vi "ReadFlowMultipleDevices Example.vi"() -> ()   [LabVIEW 2012]
uses:
  BrooksDLL.dll
panel:
  out "S2_2 String":string
  out "S1_2 String":string
  out "S2_1 String":string
  out "S1_1 String":string
  out "S2_2":u8 format="%.0x"
  out "S1_2":u8 format="%.0x"
  out "S2_1":u8 format="%.0x"
  out "S1_1":u8 format="%.0x"
  out "Function Output Comment 2":string
  out "Flow Unit String 2":string
  out "Flow Units 2":u8
  out "Flow 2":sgl format="%.2f"
  out "output param 2":i32
  out "Function Output Comment 1":string
  out "Flow Unit String 1":string
  out "Flow Units 1":u8
  out "Flow 1":sgl format="%.2f"
  out "output param 1":i32
  # "FT01"
  # "FT02"
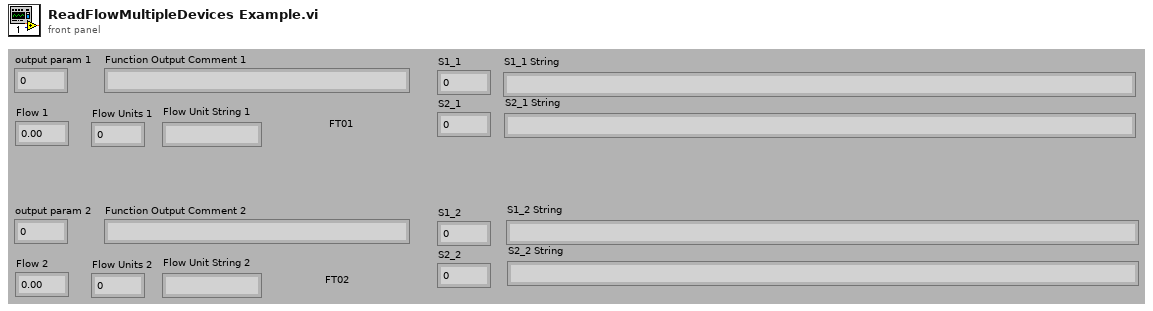
[diagram p1: front panel]
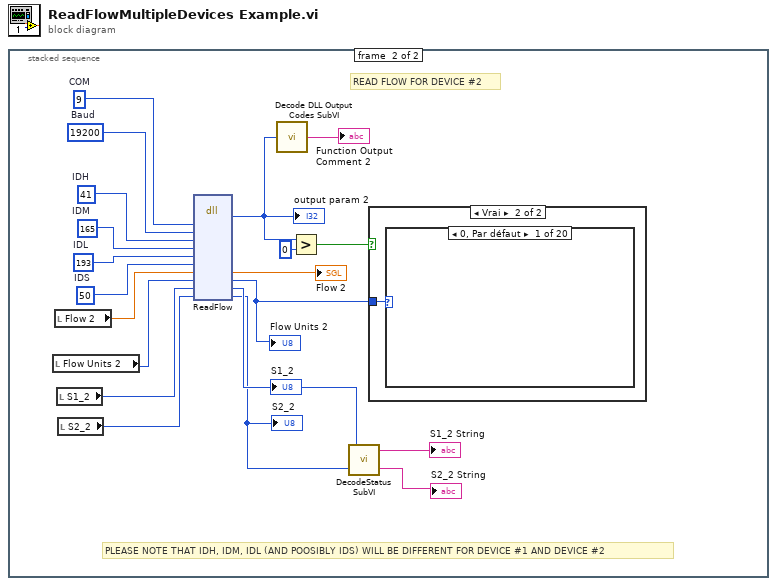
[diagram p0: block diagram]
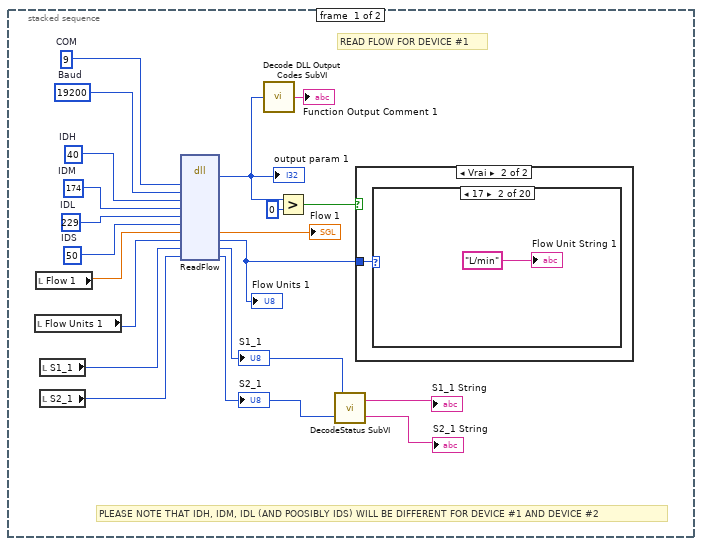
[diagram p2: hidden frame]
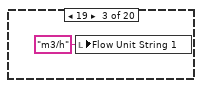
[diagram p5: hidden frame]
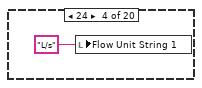
[diagram p6: hidden frame]
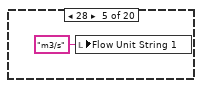
[diagram p7: hidden frame]
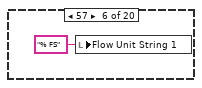
[diagram p8: hidden frame]
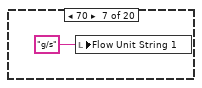
[diagram p9: hidden frame]
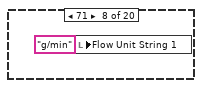
[diagram p10: hidden frame]
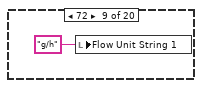
[diagram p11: hidden frame]
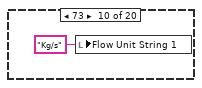
[diagram p12: hidden frame]
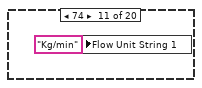
[diagram p13: hidden frame]
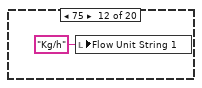
[diagram p14: hidden frame]
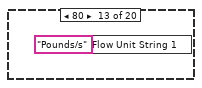
[diagram p15: hidden frame]
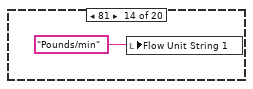
[diagram p16: hidden frame]
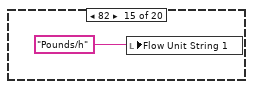
[diagram p17: hidden frame]
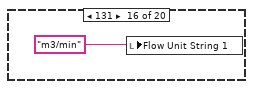
[diagram p18: hidden frame]
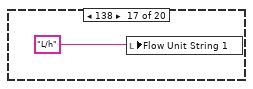
[diagram p19: hidden frame]
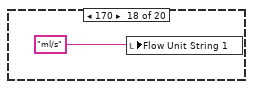
[diagram p20: hidden frame]
diagram:
  n1 = stacked-sequence {
    frame #0 {
      w15 = u8 50  # IDS
      w16 = u8 229  # IDL
      w17 = u8 174  # IDM
      w18 = u8 40  # IDH
      w19 = 19200  # Baud
      w20 = 9  # COM
      # "PLEASE NOTE THAT IDH, IDM, IDL (AND POOSIBLY IDS) WILL BE DIFFERENT FOR DEVICE #1 AND DEVICE #2"
      # "READ FLOW FOR DEVICE #1"
      n2 = local read "Flow Units 1"() -> (w10:u8)
      n3 = local read "Flow 1"() -> (w7:sgl)
      n4 = local read "S1_1"() -> (w6:u8)
      n5 = local read "S2_1"() -> (w5:u8)
      n6 = dll-call lib="C:/Users/Sylvain/Desktop/TopPerm_20150127/drivers/Brooks/S Protocol/BrooksDLL.dll" fn="ReadFlow"("COM"=w20, "Baud"=w19, "IDH"=w18, "IDM"=w17, "IDL"=w16, "IDS"=w15, "Flow"=w7, "FlowUnit"=w10, "S1"=w6, "S2"=w5) -> (w12:i32, "Flow"=→"Flow 1":sgl, "FlowUnit"=w9:u8, "S1"=w4:u8, "S2"=w3:u8)  [unwired: 9 in, 2 out]
      "output param 1" <- w12
      "Flow Units 1" <- w9
      "S1_1" <- w4
      "S2_1" <- w3
      n7 = call "Decode DLL Output Codes SubVI.vi"("Numeric"=w12) -> ("Function Output Comment"=→"Function Output Comment 1":string)
      n8 = Greater?(x=w12, y=0) -> (0:w14:bool)
      n9 = call "DecodeStatus SubVI.vi"("S2"=w3, "S1"=w4) -> ("S2 String"=→"S2_1 String":string, "S1 String"=→"S1_1 String":string)
      n10 = case shown="Vrai" w14 {
        tunnel: w9 -> [_ w21]
        frame False {
        }
        frame True {
          n11 = case shown="17" w21 {
            frame 0, Default {
            }
            frame 17 {
              "Flow Unit String 1" <- "L/min"
            }
            frame 19 {
              n12 = local write "Flow Unit String 1"("m3/h") -> ()
            }
            frame 24 {
              n13 = local write "Flow Unit String 1"("L/s") -> ()
            }
            frame 28 {
              n14 = local write "Flow Unit String 1"("m3/s") -> ()
            }
            frame 57 {
              n15 = local write "Flow Unit String 1"("% FS") -> ()
            }
            frame 70 {
              n16 = local write "Flow Unit String 1"("g/s") -> ()
            }
            frame 71 {
              n17 = local write "Flow Unit String 1"("g/min") -> ()
            }
            frame 72 {
              n18 = local write "Flow Unit String 1"("g/h") -> ()
            }
            frame 73 {
              n19 = local write "Flow Unit String 1"("Kg/s") -> ()
            }
            frame 74 {
              n20 = local write "Flow Unit String 1"("Kg/min") -> ()
            }
            frame 75 {
              n21 = local write "Flow Unit String 1"("Kg/h") -> ()
            }
            frame 80 {
              n22 = local write "Flow Unit String 1"("Pounds/s") -> ()
            }
            frame 81 {
              n23 = local write "Flow Unit String 1"("Pounds/min") -> ()
            }
            frame 82 {
              n24 = local write "Flow Unit String 1"("Pounds/h") -> ()
            }
            frame 131 {
              n25 = local write "Flow Unit String 1"("m3/min") -> ()
            }
            frame 138 {
              n26 = local write "Flow Unit String 1"("L/h") -> ()
            }
            frame 170 {
              n27 = local write "Flow Unit String 1"("ml/s") -> ()
            }
            frame 171 {
              n28 = local write "Flow Unit String 1"("ml/min") -> ()
            }
            frame 172 {
              n29 = local write "Flow Unit String 1"("ml/h") -> ()
            }
          }
        }
      }
    }
    frame #1 {
      w55 = u8 50  # IDS
      w56 = u8 193  # IDL
      w57 = u8 165  # IDM
      w58 = u8 41  # IDH
      w59 = 19200  # Baud
      w60 = 9  # COM
      # "PLEASE NOTE THAT IDH, IDM, IDL (AND POOSIBLY IDS) WILL BE DIFFERENT FOR DEVICE #1 AND DEVICE #2"
      # "READ FLOW FOR DEVICE #2"
      n30 = local read "Flow Units 2"() -> (w48:u8)
      n31 = local read "Flow 2"() -> (w47:sgl)
      n32 = local read "S1_2"() -> (w46:u8)
      n33 = local read "S2_2"() -> (w45:u8)
      n34 = dll-call lib="C:/Users/Sylvain/Desktop/TopPerm_20150127/drivers/Brooks/S Protocol/BrooksDLL.dll" fn="ReadFlow"("COM"=w60, "Baud"=w59, "IDH"=w58, "IDM"=w57, "IDL"=w56, "IDS"=w55, "Flow"=w47, "FlowUnit"=w48, "S1"=w46, "S2"=w45) -> (w51:i32, "Flow"=→"Flow 2":sgl, "FlowUnit"=w49:u8, "S1"=w44:u8, "S2"=w43:u8)  [unwired: 9 in, 2 out]
      "output param 2" <- w51
      "Flow Units 2" <- w49
      "S1_2" <- w44
      "S2_2" <- w43
      n35 = call "Decode DLL Output Codes SubVI.vi"("Numeric"=w51) -> ("Function Output Comment"=→"Function Output Comment 2":string)
      n36 = Greater?(x=w51, y=0) -> (0:w54:bool)
      n37 = call "DecodeStatus SubVI.vi"("S2"=w43, "S1"=w44) -> ("S2 String"=→"S2_2 String":string, "S1 String"=→"S1_2 String":string)
      n38 = case shown="Vrai" w54 {
        tunnel: w49 -> [_ w61]
        frame False {
        }
        frame True {
          n39 = case shown="0, Par défaut" w61 {
            frame 0, Default {
            }
            frame 17 {
              "Flow Unit String 2" <- "L/min"
            }
            frame 19 {
              n40 = local write "Flow Unit String 2"("m3/h") -> ()
            }
            frame 24 {
              n41 = local write "Flow Unit String 2"("L/s") -> ()
            }
            frame 28 {
              n42 = local write "Flow Unit String 2"("m3/s") -> ()
            }
            frame 57 {
              n43 = local write "Flow Unit String 2"("% FS") -> ()
            }
            frame 70 {
              n44 = local write "Flow Unit String 2"("g/s") -> ()
            }
            frame 71 {
              n45 = local write "Flow Unit String 2"("g/min") -> ()
            }
            frame 72 {
              n46 = local write "Flow Unit String 2"("g/h") -> ()
            }
            frame 73 {
              n47 = local write "Flow Unit String 2"("Kg/s") -> ()
            }
            frame 74 {
              n48 = local write "Flow Unit String 2"("Kg/min") -> ()
            }
            frame 75 {
              n49 = local write "Flow Unit String 2"("Kg/h") -> ()
            }
            frame 80 {
              n50 = local write "Flow Unit String 2"("Pounds/s") -> ()
            }
            frame 81 {
              n51 = local write "Flow Unit String 2"("Pounds/min") -> ()
            }
            frame 82 {
              n52 = local write "Flow Unit String 2"("Pounds/h") -> ()
            }
            frame 131 {
              n53 = local write "Flow Unit String 2"("m3/min") -> ()
            }
            frame 138 {
              n54 = local write "Flow Unit String 2"("L/h") -> ()
            }
            frame 170 {
              n55 = local write "Flow Unit String 2"("ml/s") -> ()
            }
            frame 171 {
              n56 = local write "Flow Unit String 2"("ml/min") -> ()
            }
            frame 172 {
              n57 = local write "Flow Unit String 2"("ml/h") -> ()
            }
          }
        }
      }
    }
  }
